vi "MUX - Switch Control.vi"() -> ()   [LabVIEW 2013]
doc: "Sample numeric display item."
uses:
  <vilib>/NI Veristand/Display Template Support/Display Template Support.llb/cluster_Screen Item Settings.ctl
  <vilib>/NI Veristand/Display Template Support/Display Template Support.llb/cluster_Graph Scale Settings.ctl
  <vilib>/NI Veristand/Display Template Support/Display Template Support.llb/cluster_Graph Plot Settings.ctl
  NationalInstruments.VeriStand.SystemStorage
  SubVIs/Relay Data.ctl
  SubVIs/Switch.ctl
  <vilib>/NI Veristand/Display Template Support/Display Template Support.llb/enum_Display Template Handler Minimal To Widget Msg.ctl
  <vilib>/NI Veristand/Display Template Support/Display Template Support.llb/enum_Display Template Handler Minimal To Workspace.ctl
  <vilib>/NI Veristand/Display Template Support/Display Template Support.llb/sub_Display Template Handler Custom.vi
  <vilib>/NI Veristand/Execution/Workspace/NI_VS Workspace ExecutionAPI.lvlib
  MUX Custom Device.lvlib
panel:
  in  "NIVS.Gateway IP Address":string
  in  "Open":bool
  in  "Relays":T1[](array[typedef])
  in  "NIVS.System Definition Root":refnum<k24>
  in  "Item.Data":T3
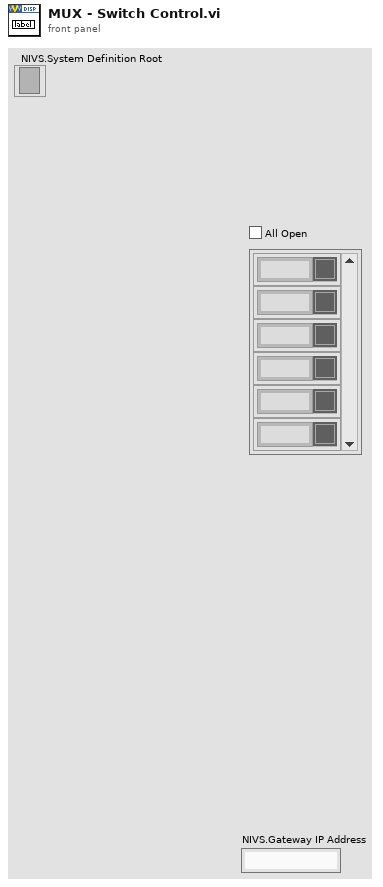
[diagram p1: front panel]
types:
  T1 = typedef "MUX Custom Device.lvlib/Relay Data.ctl" = cluster{"Relay Name":string, "State":T2}
  T2 = typedef "MUX Custom Device.lvlib/Switch.ctl" = bool
  T3 = typedef "cluster_Screen Item Settings.ctl" = cluster{"Template VI":string, "Position X":i32, "Position Y":i32, "Custom":string, "Show Title Bar":bool, "ID":i32, "Always On Top":bool, "Allow Resize":bool, "Allow Minimize":bool, "Allow Close":bool, "Size to Screen":bool, "Screen.ID":i32, "State":enum16{"Normal", "New"}, "Title":string, "Window Bounds":cluster{"[0]":i16, "[1]":i16, "[2]":i16, "[3]":i16}, "Channel Ref":u64, "Unit":string, "Default Units?":bool, "Flash Limit?":bool, "Color 1":u32, "Color 2":u32, "Color 3":u32, "Color 4":u32, "Bck Color":u32, "Fore Color":u32, "Limit 1":dbl, "Limit 2":dbl, "Limit 3":dbl, "Limit 4":dbl, "Limit Mode 1":i32, "Limit Mode 2":i32, "Limit Mode 3":i32, "Limit Mode 4":i32, "Scale Precision":i32, "Scale Min":dbl, "Scale Max":dbl, "Format":i32, "Precision":i32, "Background Type":i32, "IDs":i32[], "Units":string[], "Labels":string[], "Scale Factor":dbl, "Scale Offset":dbl, "YScale Index":u32[], "XScale":T4, "YScales":T4[], "Plots":T5[], "Update Period":dbl, "History Length":dbl, "My.Ref":refnum<vi>, "Is Control?":bool, "Channel Paths":string[], "Custom Data":variant}
  T4 = typedef "cluster_Graph Scale Settings.ctl" = cluster{"Format":u8, "Precision":u8, "Fit":u8, "Label":string, "Use Default Label":bool, "Label Visible":bool, "Min":dbl, "Max":dbl}
  T5 = typedef "cluster_Graph Plot Settings.ctl" = cluster{"Bar Style":u8, "Fill To":i16, "Fill/PtColor":u32, "Line Style":u8, "Line Width":u8, "Color":u32, "Interp":u8, "Point Style":u8}
  T6 = typedef "enum_Display Template Handler Minimal To Workspace.ctl" = cluster{"Operation":enum16{"SetCustomData", "DeleteItem"}, "Data":variant}
  T7 = typedef "enum_Display Template Handler Minimal To Widget Msg.ctl" = enum16{"Stop", "LaunchConfigDialog"}
  T8 = typedef "NI_VS Workspace ExecutionAPI.lvlib/WorkspaceAPI.ctl" = refnum<k24>
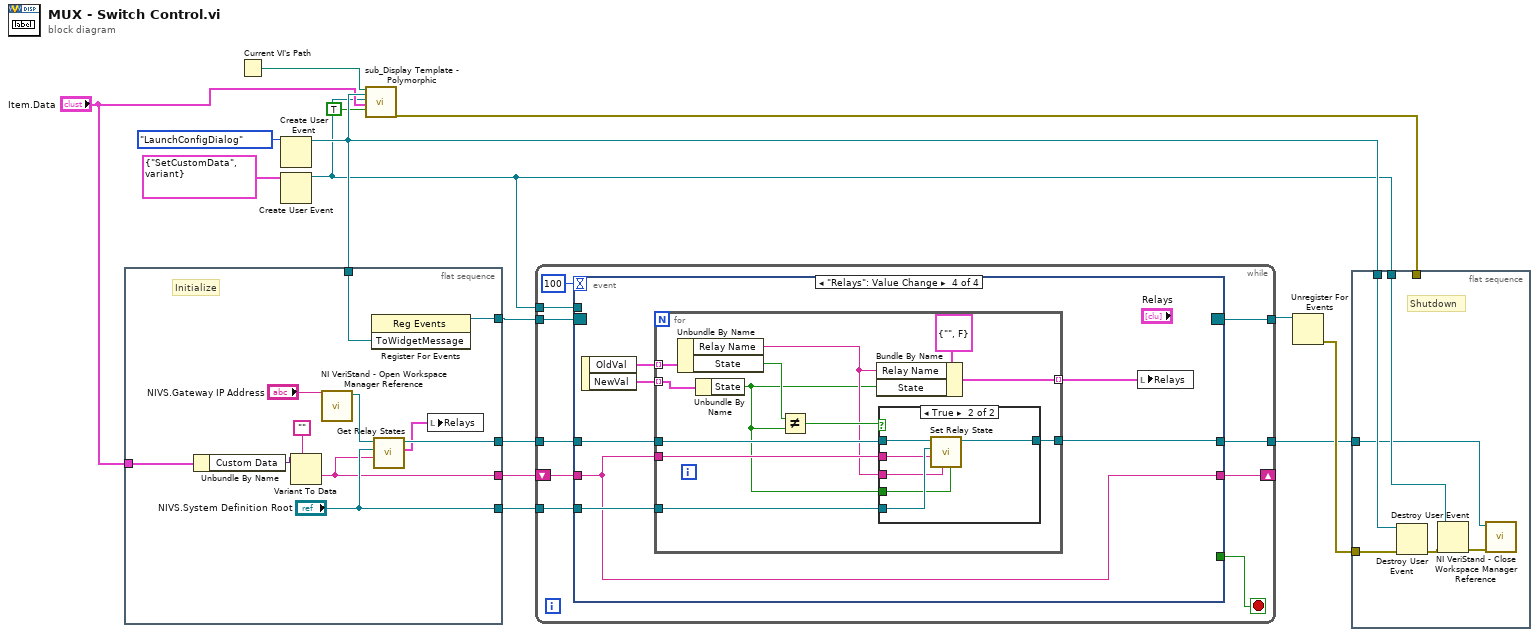
[diagram p0: block diagram]
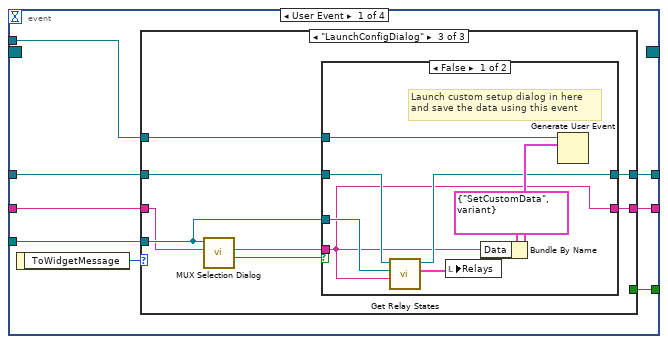
[diagram p2: hidden frame]
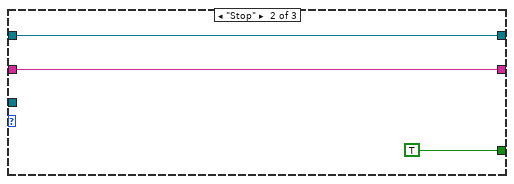
[diagram p4: hidden frame]
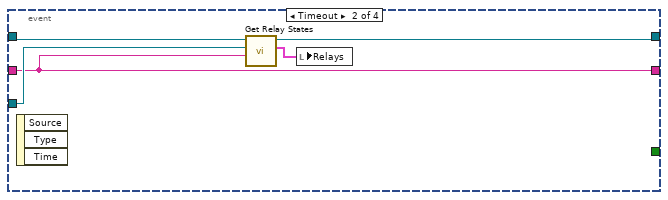
[diagram p6: hidden frame]
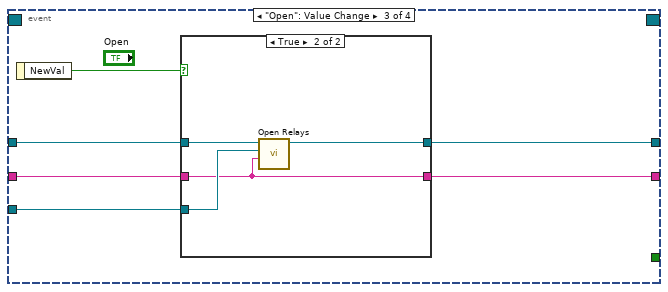
[diagram p7: hidden frame]
diagram:
  n1 = flat-sequence {
    tunnel: [w26] -> w13
    tunnel: w10 -> [w25]
    tunnel: "Item.Data" -> [w24]
    tunnel: ["NIVS.System Definition Root"] -> w4
    tunnel: [w17] -> w3
    tunnel: [w19] -> w2
    frame #0 {
      # "Initialize"
      n2 = Unbundle By Name(w24) -> ("Custom Data"=w23:variant)
      n3 = Variant To Data(type="", Variant=w23) -> (data=w17:string)  [unwired: 1 in, 1 out]
      n4 = call <vilib>:"NI VeriStand - Open Workspace Manager Reference.vi"("Gateway IP Address (\"\": localhost)"="NIVS.Gateway IP Address") -> ("WorkspaceManager"=w20:T8)  [unwired: 9 in, 1 out]
      n5 = register-events(w25) -> (reference out=w26:refnum<event-registration>)  [unwired: 2 in, 1 out]
      n6 = call "Get Relay States.vi"("nodePath"=w17, "NIVS.System Definition Root"="NIVS.System Definition Root", "WorkspaceManager in"=w20) -> ("Relays"=w16:T1[], "WorkspaceManager out"=w19:T8)  [unwired: 6 in, 1 out]
      n7 = local write "Relays"(w16) -> ()
    }
  }
  n8 = Current VI's Path() -> (path=w8:path)
  n9 = Create User Event(user event datatype=enum_Display_Template_Handler_Minimal_To_Widget_Msg."LaunchConfigDialog" ("ToWidgetMessage")) -> (user event=w10:refnum<user-event>)  [unwired: 1 in, 1 out]
  n10 = Create User Event(user event datatype=T6 {"Operation"=enum."SetCustomData", "Data"=variant} ("Data")) -> (user event=w6:refnum<user-event>)  [unwired: 1 in, 1 out]
  n11 = call-poly <vilib>:"sub_Display Template - Polymorphic.vi"("Parent.Path"=w8, "ToWidgetEvent"=w10, "ToWorkspace"=w6, "Item.Data"="Item.Data", "Resizable"=TRUE) -> ("error out"=w15:errorcluster)  [unwired: 1 in, 13 out]
  n12 = while {
    tunnel: w13 -> [w36]
    tunnel: [w34] -> w12
    tunnel: w6 -> [w33]
    tunnel: w4 -> [w32]
    tunnel: w2 -> [w30]
    tunnel: [w29] -> w1
    shift-right: [w27] -> _
    shift-left: w3 -> [w31]
    stop <- w35 stop-if-true
    n13 = event shown="[3] \"Relays\": Value Change" {
      selector: w36 -> [_ _ _ _]
      dyn-events: [_ _ _ _] -> w34
      timeout: 100 -> [_ _ _ _]
      tunnel: [w43 _ _ _] -> w35
      tunnel: w33 -> [w42 _ _ _]
      tunnel: w32 -> [w41 w71 w76 w87]
      tunnel: w31 -> [w40 w68 w75 w86]
      tunnel: w30 -> [w39 w72 w77 w88]
      tunnel: [w38 w70 w74 w85] -> w29
      tunnel: [w37 w68 w73 w86] -> w27
      event User Event {
        n14 = event-data() -> ("ToWidgetMessage"=w44:T7)  [unwired: 1 out]
        n15 = case shown="\"LaunchConfigDialog\"" w44 {
          tunnel: [_ TRUE _] -> w43
          tunnel: w42 -> [_ _ w57]
          tunnel: w41 -> [_ _ w54]
          tunnel: w40 -> [w45 w47 w50]
          tunnel: w39 -> [w46 w48 w53]
          tunnel: [w46 w48 w52] -> w38
          tunnel: [w45 w47 w51] -> w37
          frame Default {
          }
          frame "Stop" {
          }
          frame "LaunchConfigDialog" {
            n16 = call "MUX Selection Dialog.vi"("Current selection"=w50, "NIVS.System Definition Root"=w54) -> ("Cancelled"=w55:bool, "New selection"=w56:string)  [unwired: 7 in, 1 out]
            n17 = case shown="False" w55 {
              tunnel: w57 -> [w65 _]
              tunnel: w56 -> [w58 w66]
              tunnel: w54 -> [w62 _]
              tunnel: w53 -> [w61 w67]
              tunnel: [w59 w67] -> w52
              tunnel: [w58 w66] -> w51
              frame False {
                # "Launch custom setup dialog in here\nand save the data using this event"
                n18 = call "Get Relay States.vi"("nodePath"=w58, "NIVS.System Definition Root"=w62, "WorkspaceManager in"=w61) -> ("Relays"=w60:T1[], "WorkspaceManager out"=w59:T8)  [unwired: 6 in, 1 out]
                n19 = local write "Relays"(w60) -> ()
                n20 = Bundle By Name(cluster=T6 {"Operation"=enum."SetCustomData", "Data"=variant} ("event data"), "Data"=w58) -> (w63:T6)
                n21 = Generate User Event(user event=w65, event data cluster=w63) -> ()  [unwired: 2 in, 2 out]
              }
              frame True {
              }
            }
          }
        }
      }
      event Timeout {
        n22 = event-data() -> ()  [unwired: 4 out]
        n23 = call "Get Relay States.vi"("nodePath"=w68, "NIVS.System Definition Root"=w71, "WorkspaceManager in"=w72) -> ("Relays"=w69:T1[], "WorkspaceManager out"=w70:T8)  [unwired: 6 in, 1 out]
        n24 = local write "Relays"(w69) -> ()
      }
      event "Open": Value Change {
        n25 = event-data() -> ("NewVal"=w78:bool)  [unwired: 1 out]
        n26 = case shown="True" w78 {
          tunnel: w77 -> [w80 w84]
          tunnel: w76 -> [_ w83]
          tunnel: w75 -> [w79 w81]
          tunnel: [w80 w82] -> w74
          tunnel: [w79 w81] -> w73
          frame False {
          }
          frame True {
            n27 = call "Open Relays.vi"("nodePath"=w81, "NIVS.System Definition Root"=w83, "WorkspaceManager in"=w84) -> ("WorkspaceManager out"=w82:T8)  [unwired: 7 in, 1 out]
          }
        }
      }
      event "Relays": Value Change {
        n28 = event-data() -> ("OldVal"=w90:T1[], "NewVal"=w91:T1[])  [unwired: 1 out]
        n29 = for {
          tunnel: w91 -> [w102] mode=indexing
          tunnel: w90 -> [w103] mode=indexing
          tunnel: [w99] -> w89 mode=indexing
          tunnel: w88 -> [w97]
          tunnel: w87 -> [w96]
          tunnel: w86 -> [w95]
          tunnel: [w92] -> w85
          n30 = Unbundle By Name(w103) -> ("Relay Name"=w94:string, "State"=w101:T2)
          n31 = Unbundle By Name(w102) -> ("State"=w93:T2)
          n32 = Not Equal?(x=w101, y=w93) -> (x != y?=w98:T2)
          n33 = Bundle By Name(cluster=T1 {"Relay Name"="", "State"=FALSE} ("Relay Data"), "Relay Name"=w94, "State"=w93) -> (w99:T1)
          n34 = case shown="True" w98 {
            tunnel: w97 -> [w104 w110]
            tunnel: w96 -> [_ w109]
            tunnel: w95 -> [_ w108]
            tunnel: w94 -> [_ w107]
            tunnel: w93 -> [_ w106]
            tunnel: [w104 w105] -> w92
            frame False {
            }
            frame True {
              n35 = call "Set Relay State.vi"("State"=w106, "Relay Name"=w107, "nodePath"=w108, "NIVS.System Definition Root"=w109, "WorkspaceManager in"=w110) -> ("WorkspaceManager out"=w105:T8)  [unwired: 5 in, 1 out]
            }
          }
        }
        n36 = local write "Relays"(w89) -> ()
      }
    }
  }
  n37 = Unregister For Events(event registration refnum=w12) -> (error out=w11:errorcluster)  [unwired: 1 in]
  n38 = flat-sequence {
    tunnel: w15 -> [_]
    tunnel: w11 -> [w115]
    tunnel: w10 -> [w116]
    tunnel: w6 -> [w113]
    tunnel: w1 -> [w111]
    frame #0 {
      # "Shutdown"
      n39 = Destroy User Event(user event=w116, error in=w115) -> (error out=w114:errorcluster)
      n40 = Destroy User Event(user event=w113, error in=w114) -> (error out=w112:errorcluster)
      n41 = call <vilib>:"NI VeriStand - Close Workspace Manager Reference.vi"("error in (no error)"=w112, "WorkspaceManager"=w111) -> ()  [unwired: 9 in, 1 out]
    }
  }
